vi "Log.Debug.vi"(8 "error in":errorcluster, 9 "Append newline? (T)":bool=TRUE, 10 "Add to log file? (F)":bool, 11 "Message":string) -> (0 "error out":errorcluster)   [LabVIEW 2026, in "SystemMonitor Engine.lvlib" / "SystemMonitor Engine.lvclass"]
uses:
  SystemMonitor Engine.lvclass
  SystemMonitor Engine.lvclass/SystemMonitor Engine.ctl
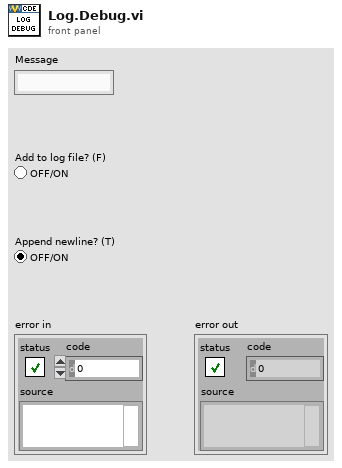
[diagram p1: front panel]
types:
  T1 = cluster{"Message":string, "Level":enum16{"Error", "Warning", "Info", "Debug"}, "Add to log file? (F)":bool, "Append newline? (T)":bool}
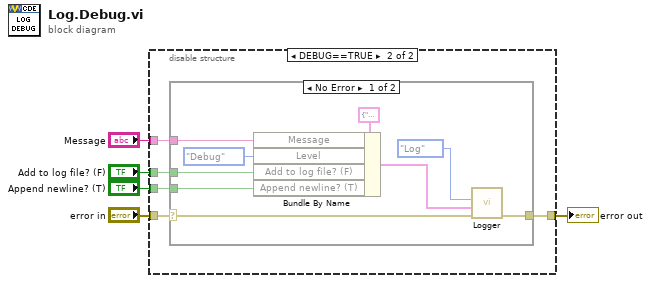
[diagram p0: block diagram]
diagram:
  n1 = disable-structure shown="DEBUG==TRUE" {
    disable-tunnel: "error in" -> [w6 w11]
    disable-tunnel: [w6 w10] -> w4
    disable-tunnel: "Message" -> [_ w9]
    disable-tunnel: "Add to log file? (F)" -> [_ w8]
    disable-tunnel: "Append newline? (T)" -> [_ w7]
    frame condition #0 (active) {
    }
    frame condition #1 {
      n2 = case shown="No Error" w11 {
        selector: w11 -> [w20 w21]
        tunnel: w9 -> [w17 _]
        tunnel: w8 -> [w15 _]
        tunnel: w7 -> [w14 _]
        tunnel: [w19 w21] -> w10
        frame No Error {
          n3 = Bundle By Name(cluster=T1 {"Message"="", "Level"=enum."Error", "Add to log file? (F)"=FALSE, "Append newline? (T)"=TRUE} ("Log"), "Message"=w17, "Level"=enum16{"Error", "Warning", "Info", "Debug"}."Debug", "Add to log file? (F)"=w15, "Append newline? (T)"=w14) -> (w12:T1)
          n4 = call "Logger.vi"("error in"=w20, "Log"=w12, "State"=enum16{"Initialize", "Log"}."Log") -> ("error out"=w19:errorcluster)  [unwired: 7 in, 1 out]
        }
        frame Error {
        }
      }
    }
  }
  "error out" <- w4
